vi "Process.vi"(8 "error in (no error)":errorcluster, 10 "Pound in":refnum<class "Pound.lvclass">, 11 "Qbus in":refnum<class "Qbus.lvclass">) -> (0 "error out":errorcluster)   [LabVIEW 2017, in "McsaFpgaAcquisition.lvlib"]
doc: "Acquires waveforms from channels on NI 9242 and NI 9239 C Series modules. This process transfers data from a device-specific FPGA bitfile that reads samples directly from the FPGA at the sampling rate configured for the device."
uses:
  <vilib>/addons/InsightCM/Devices/Shared/Mcsa/McsaFpgaAcquisition/McsaFpgaAcquisition.lvlib
  <vilib>/addons/Qbus/Qbus.lvclass
  <vilib>/NI/Software Watchdog/Pound/Pound.lvclass
  <vilib>/addons/InsightCM/Devices/Shared/Cms/CmsAcquisition/controls/State.ctl
  <vilib>/addons/InsightCM/Devices/Shared/Mcsa/McsaFpgaAcquisition/controls/Configuration.ctl
  <vilib>/addons/InsightCM/Devices/Shared/Cms/CmsAcquisition/controls/FixedSizeArrays.ctl
  <vilib>/LabVIEW Targets/FPGA/cRIO/shared/nicrio_ModuleControls/nicrio_cRIO-9232_ConfigModeRing.ctl
  <vilib>/addons/InsightCM/Devices/Shared/Cms/cRIOWfmAcq/subVIs/RIO Wfm Cust Ctrls/rwfm_SamplingInfo.ctl
  <vilib>/addons/InsightCM/Devices/Shared/Mcsa/McsaFpgaAcquisition/controls/Group.ctl
  <vilib>/addons/InsightCM/Devices/Shared/Mcsa/McsaFpgaAcquisition/controls/ChannelMcsa.ctl
  <vilib>/addons/InsightCM/Devices/Shared/Mcsa/McsaFpgaAcquisition/controls/RangeParams.ctl
  <vilib>/addons/InsightCM/Devices/Shared/Common/DataFlow/controls/Type.ctl
  <vilib>/addons/InsightCM/Devices/Shared/Cms/cRIOWfmAcq/cRIOWfmLib.lvlib
  <vilib>/NI/Software Watchdog/Watchdog/Watchdog.lvclass
  <vilib>/addons/InsightCM/Devices/Shared/Common/FpgaBitfileManager/FpgaBitfileManager.lvlib
  <vilib>/addons/InsightCM/Devices/Shared/Common/DataFlow/DataFlow.lvlib
  <vilib>/addons/InsightCM/Utilities/GlobalConfiguration/GlobalConfiguration.lvlib
  <vilib>/addons/InsightCM/Devices/Shared/Common/ServerComm/ServerComm.lvlib
  <vilib>/addons/InsightCM/Devices/Shared/Mcsa/cRIOWfmAcqMcsa/cRIOWfmLibMcsa.lvlib
  <vilib>/addons/InsightCM/Devices/Shared/Mcsa/McsaDataEventCreator/McsaDataEventCreator.lvlib
  <vilib>/addons/TraceLogger/TraceLogger.lvlib
  <vilib>/addons/InsightCM/Devices/Shared/Cms/CmsAcquisition/CmsAcquisition.lvlib
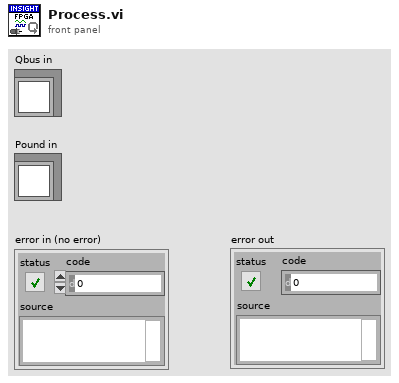
[diagram p1: front panel]
types:
  T1 = typedef "McsaFpgaAcquisition.lvlib/Configuration.ctl" = cluster{"NumberOfModules":i16, "Dynamic FPGA VI Ref":refnum<k20>, "FixedSizeX31":T2, "SamplingInfo":T4, "BlockSize (sec)":dbl, "Samples To Read (per chan)":i32, "RunningAcquisitionLength":dbl, "Settling Time":dbl, "Waveform Groups":T5[], "Acquisition Block Number":i32, "Device Name":string, "ValidConfig":bool, "delta connection?":bool}
  T2 = typedef "CmsAcquisition.lvlib/FixedSizeArrays.ctl" = cluster{"EnabledChannels":bool[], "Sensitivity":dbl[], "InputConfig":T3[]}
  T3 = typedef "nicrio_cRIO-9232_ConfigModeRing.ctl" = u8
  T4 = typedef "cRIOWfmLib.lvlib/rwfm_SamplingInfo.ctl" = cluster{"Number of Channels":i32, "Sampling Rate":dbl, "Channels":string[], "Units":string[], "Offsets":sgl[]}
  T5 = typedef "McsaFpgaAcquisition.lvlib/Group.ctl" = cluster{"Name":string, "Channels":T6[]}
  T6 = typedef "McsaFpgaAcquisition.lvlib/ChannelMcsa.ctl" = cluster{"Name":string, "Status Tag":string, "RangeCheck":T7}
  T7 = typedef "McsaFpgaAcquisition.lvlib/RangeParams.ctl" = cluster{"Enabled":bool, "Max":dbl, "Min":dbl}
  T8 = typedef "CmsAcquisition.lvlib/State.ctl" = enum16{"Unconfigured", "Configured", "Acquiring", "Stopped", "BurstMode"}
  T9 = typedef "DataFlow.lvlib/Type.ctl" = enum16{"High Rate", "Low Rate", "Burst Mode"}
  T10 = typedef "McsaDataEventCreator.lvlib/RegisterDataSets.ctl" = cluster{"DataGroup":string, "DataSets":T11[]}
  T11 = typedef "McsaDataEventCreator.lvlib/Registry_DataSet.ctl" = cluster{"ChannelName":string, "DataSetType":T12, "DoNotWriteToDB":bool, "ParentName":string}
  T12 = typedef "McsaDataEventCreator.lvlib/DataSetType.ctl" = enum16{"Waveform", "MCSAFFT", "TorqueWFM"}
  T13 = typedef "DataFlow.lvlib/Data.ctl" = cluster{"DataGroup":string, "Waveforms":T14, "Map":T15, "Type":T9}
  T14 = typedef "wfmSGL_DVR.ctl" = refnum<data-value>
  T15 = typedef "PointValueMap.lvlib/PointMap.ctl" = refnum<data-value>
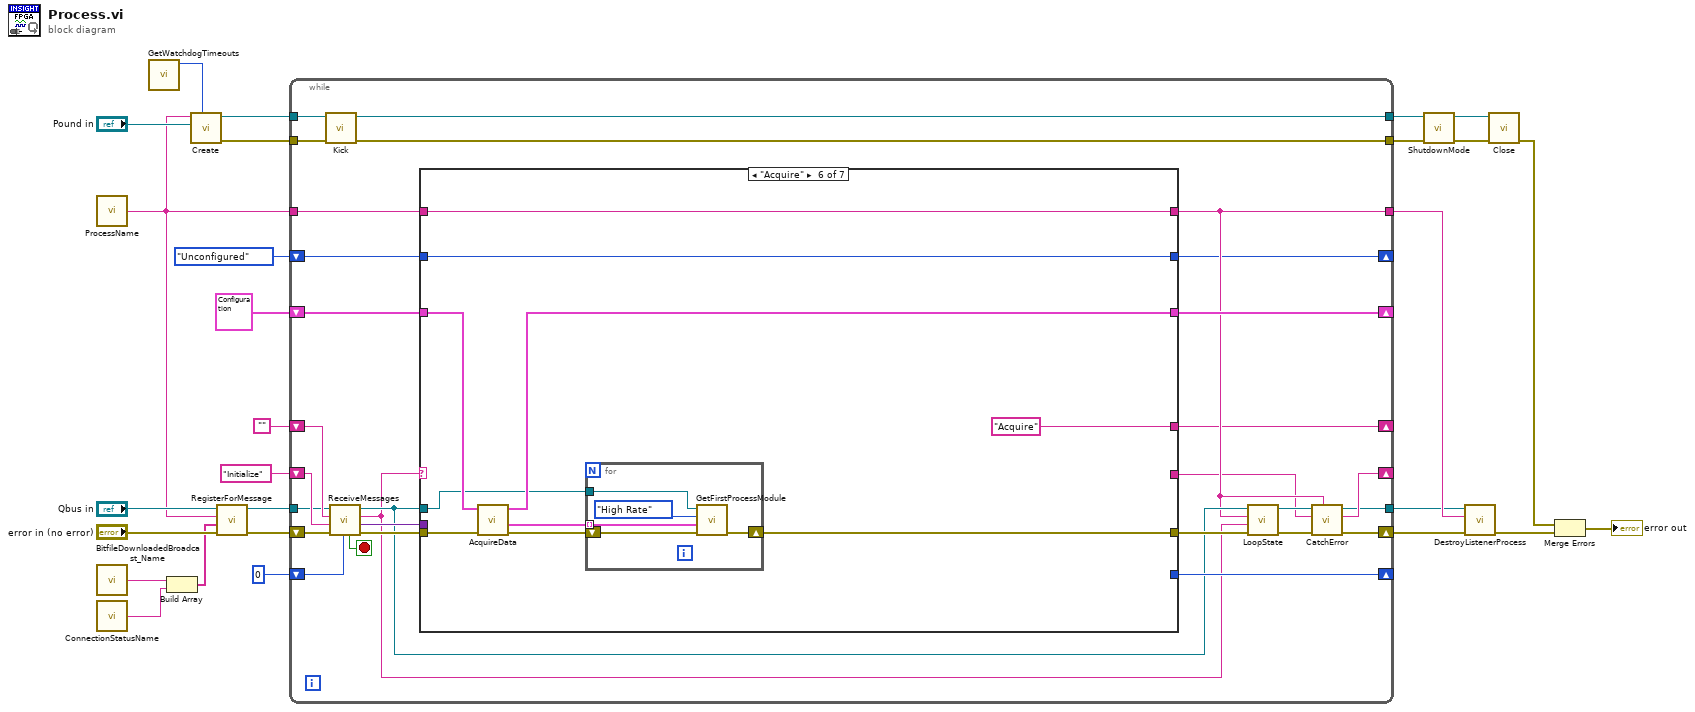
[diagram p0: block diagram]
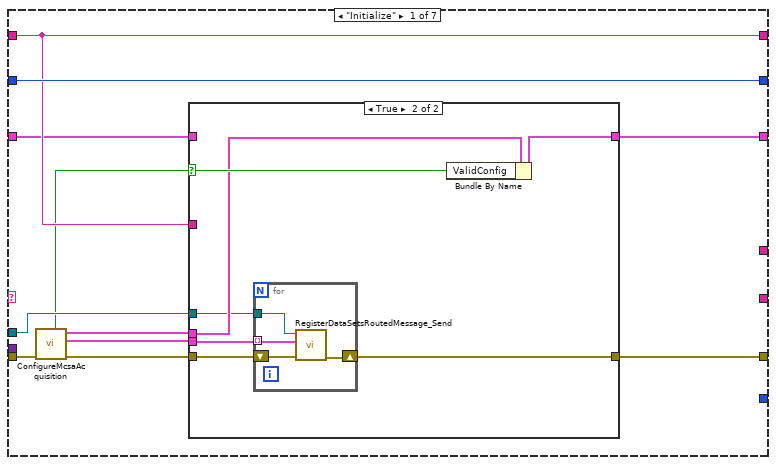
[diagram p2: hidden frame]
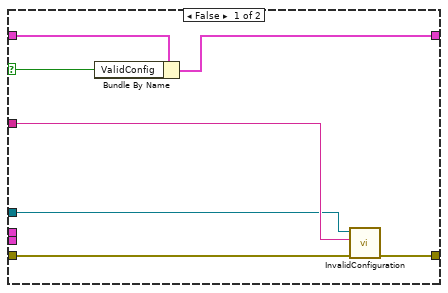
[diagram p3: hidden frame]
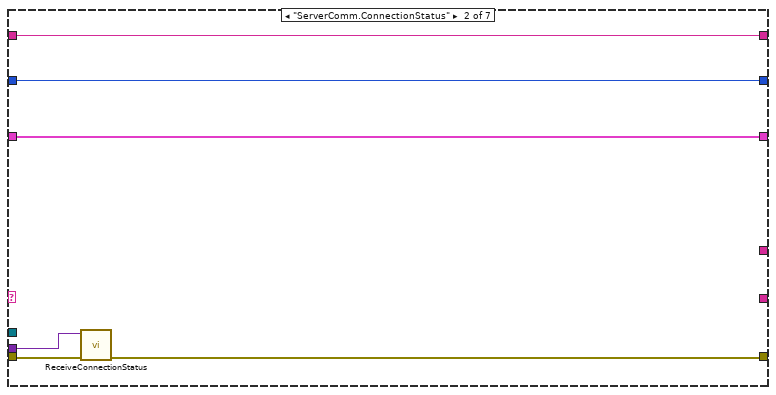
[diagram p4: hidden frame]
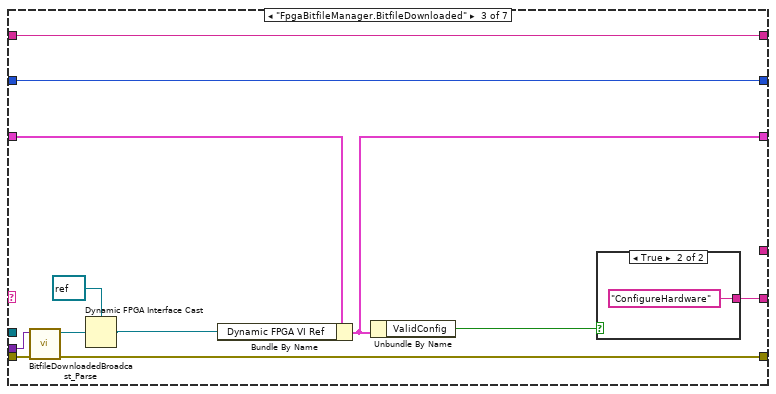
[diagram p5: hidden frame]
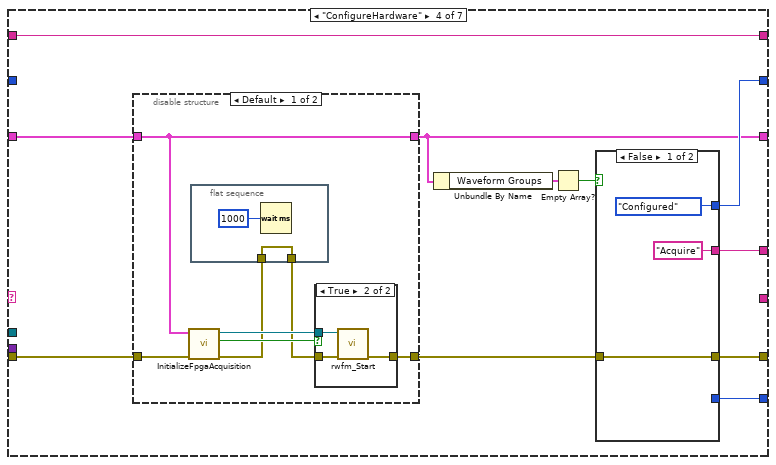
[diagram p7: hidden frame]
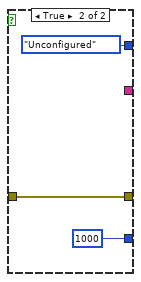
[diagram p8: hidden frame]
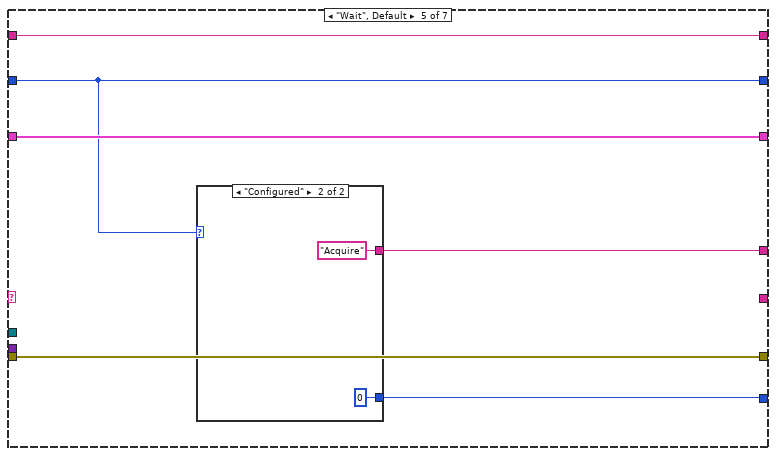
[diagram p11: hidden frame]
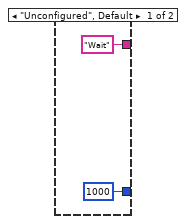
[diagram p12: hidden frame]
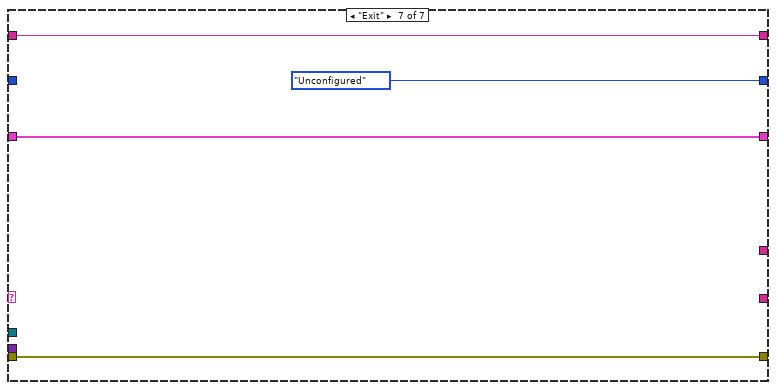
[diagram p13: hidden frame]
diagram:
  n1 = call <vilib>:"ProcessName.vi"() -> ("process name"=w4:string)  [unwired: 5 in]
  n2 = call <vilib>:"BitfileDownloadedBroadcast_Name.vi"() -> ("message name"=w9:string)  [unwired: 5 in]
  n3 = call <vilib>:"ConnectionStatusName.vi"() -> ("message name"=w1:string)  [unwired: 5 in]
  n4 = call <vilib>:"GetWatchdogTimeouts.vi"() -> ("software timeout"=w2:u32)  [unwired: 10 in, 1 out]
  n5 = Build Array(w9, w1) -> (w10:string[])
  n6 = call <vilib>:"Create.vi"("Execution Timeout (ms)"=w2, "Pound"="Pound in", "Name"=w4) -> ("error out"=w23:errorcluster, "Watchdog"=w24:refnum<data-value>)  [unwired: 7 in]
  n7 = call <vilib>:"RegisterForMessage.vi"("error in (no error)"="error in (no error)", "message names"=w10, "process name"=w4, "Qbus in"="Qbus in") -> ("error in (no error)"=w12:errorcluster, "Qbus out"=w13:refnum<class "Qbus.lvclass">)  [unwired: 6 in]
  n8 = while {
    shift-right: [w44] -> w5
    shift-left: w12 -> [w51]
    shift-right: [w34] -> _
    shift-left: "" -> [w53]
    shift-right: [w56] -> _
    shift-left: T1 {"NumberOfModules"=0, "Dynamic FPGA VI Ref"=refnum, "FixedSizeX31"={"EnabledChannels"=[], "Sensitivity"=[], "InputConfig"=[]}, "SamplingInfo"={"Number of Channels"=0, "Sampling Rate"=0.0, "Channels"=[], "Units"=[], "Offsets"=[]}, "BlockSize (sec)"=0.0, "Samples To Read (per chan)"=0, "RunningAcquisitionLength"=0.0, "Settling Time"=0.0, "Waveform Groups"=[], "Acquisition Block Number"=0, "Device Name"="", "ValidConfig"=FALSE, "delta connection?"=FALSE} ("MCSA Acquisition Configuration") -> [w28]
    shift-right: [w32] -> _
    shift-left: State."Unconfigured" ("loop state") -> [w55]
    shift-right: [w54] -> _
    shift-left: 0 ("milliseconds to wait") -> [w49]
    shift-right: [w42] -> _
    shift-left: "Initialize" -> [w52]
    tunnel: w13 -> [w50]
    tunnel: w4 -> [w29]
    tunnel: [w40] -> w6
    tunnel: [w35] -> w26
    tunnel: w24 -> [w39]
    tunnel: w23 -> [w38]
    tunnel: [w37] -> w20
    tunnel: [w36] -> w19
    stop <- w30 stop-if-true
    n9 = call <vilib>:"Kick.vi"("error in (no error)"=w38, "Watchdog"=w39) -> ("error out"=w36:errorcluster, "Watchdog"=w37:refnum<data-value>)  [unwired: 8 in]
    n10 = call <vilib>:"ReceiveMessages.vi"("timeout(100)"=w49, "error in (no error)"=w51, "priority action"=w52, "default action"=w53, "qbus in"=w50) -> ("error out"=w48:errorcluster, "msg value"=w47:variant, "action"=w31:string, "qbus out"=w43:refnum<class "Qbus.lvclass">, "exit"=w30:bool)  [unwired: 2 in]
    n11 = case shown="\"Acquire\"" w31 {
      tunnel: w48 -> [w65 w90 w95 w114 w142 w149 w162]
      tunnel: [w62 w89 w94 w111 w142 w148 w162] -> w45
      tunnel: [_ _ _ w110 w140 "Acquire" _] -> w34
      tunnel: [w57 w86 w93 w106 w141 w152 w165] -> w56
      tunnel: w28 -> [w58 w86 w102 w115 w141 w153 w165]
      tunnel: w55 -> [w63 w88 w98 _ w137 w151 _]
      tunnel: [_ _ _ w105 w138 _ _] -> w54
      tunnel: w29 -> [w60 w91 w103 w113 w139 w150 w163]
      tunnel: w47 -> [_ w87 w96 _ _ _ _]
      tunnel: w43 -> [w64 _ _ _ _ w147 _]
      tunnel: [w60 w91 w103 w113 w139 w150 w163] -> w35
      tunnel: [_ _ w99 _ _ _ _] -> w33
      tunnel: [w63 w88 w98 w109 w137 w151 State."Unconfigured" ("loop state")] -> w32
      frame "Initialize" {
        n12 = call <vilib>:"ConfigureMcsaAcquisition.vi"("error in (no error)"=w65) -> ("error out"=w67:errorcluster, "register data sets"=w66:T10[], "Mcsa Acquisition Config"=w61:T1, "valid"=w59:bool)  [unwired: 7 in]
        n13 = case shown="True" w59 {
          selector: w59 -> [w70 w77]
          tunnel: w67 -> [w68 w81]
          tunnel: w66 -> [_ w80]
          tunnel: w64 -> [w69 w75]
          tunnel: [w74 w79] -> w62
          tunnel: w61 -> [_ w76]
          tunnel: w60 -> [w73 _]
          tunnel: w58 -> [w72 _]
          tunnel: [w71 w78] -> w57
          frame False {
            n14 = Bundle By Name(cluster=w72, "ValidConfig"=w70) -> (w71:T1)
            n15 = call <vilib>:"InvalidConfiguration.vi"("error in (no error)"=w68, "description"=w73, "Qbus in"=w69) -> ("error out"=w74:errorcluster)  [unwired: 7 in, 1 out]
          }
          frame True {
            n16 = for {
              shift-right: [w84] -> w79
              shift-left: w81 -> [w85]
              tunnel: w80 -> [w82] mode=indexing
              tunnel: w75 -> [w83]
              n17 = call <vilib>:"RegisterDataSetsRoutedMessage_Send.vi"("error in (no error)"=w85, "RegisterDataSet"=w82, "Qbus in"=w83) -> ("error out"=w84:errorcluster)  [unwired: 7 in, 1 out]
            }
            n18 = Bundle By Name(cluster=w76, "ValidConfig"=w77) -> (w78:T1)
          }
        }
      }
      frame "ServerComm.ConnectionStatus" {
        n19 = call <vilib>:"ReceiveConnectionStatus.vi"("error in (no error)"=w90, "body"=w87) -> ("error out"=w89:errorcluster)  [unwired: 6 in, 3 out]
      }
      frame "FpgaBitfileManager.BitfileDownloaded" {
        n20 = call <vilib>:"BitfileDownloadedBroadcast_Parse.vi"("error in (no error)"=w95, "data"=w96) -> ("error out"=w94:errorcluster, "FPGA reference"=w97:refnum<k20>)  [unwired: 8 in]
        n21 = Dynamic FPGA Interface Cast(Session In=refnum<k20> refnum ("Dynamic FPGA VI Ref"), Type=w97) -> (Session Out=w101:refnum<k20>)
        n22 = Bundle By Name(cluster=w102, "Dynamic FPGA VI Ref"=w101) -> (w93:T1)
        n23 = Unbundle By Name(w93) -> ("ValidConfig"=w92:bool)
        n24 = case shown="True" w92 {
          tunnel: [_ "ConfigureHardware"] -> w99
          frame False {
          }
          frame True {
          }
        }
      }
      frame "ConfigureHardware" {
        n25 = disable-structure shown="Default" {
          disable-tunnel: w115 -> [w125 w135]
          disable-tunnel: w114 -> [w128 w136]
          disable-tunnel: [w127 w136] -> w112
          disable-tunnel: [w125 w135] -> w106
          frame condition #0 (active) {
            n26 = call <vilib>:"InitializeFpgaAcquisition.vi"("error in (no error)"=w128, "MCSA Acquisition Config"=w125) -> ("error out"=w123:errorcluster, "start acquisition?"=w124:bool, "dynamic FPGA VI reference"=w126:refnum<k20>)  [unwired: 7 in]
            n27 = flat-sequence {
              tunnel: [w129] -> w122
              tunnel: w123 -> [w129]
              frame #0 {
                n28 = Wait (ms)(milliseconds to wait=u32 1000) -> ()  [unwired: 1 out]
              }
            }
            n29 = case shown="True" w124 {
              tunnel: [w131 w134] -> w127
              tunnel: w122 -> [w131 w133]
              tunnel: w126 -> [_ w132]
              frame False {
              }
              frame True {
                n30 = call <vilib>:"rwfm_Start.vi"("error in"=w133, "Dynamic FPGA VI Reference"=w132) -> ("error out"=w134:errorcluster)  [unwired: 7 in, 2 out]
              }
            }
          }
          frame condition #1 {
            # "user could add simulated hardware here for MCSA device"
          }
        }
        n31 = Unbundle By Name(w106) -> ("Waveform Groups"=w108:T5[])
        n32 = Empty Array?(array=w108) -> (empty?=w107:bool)
        n33 = case shown="False" w107 {
          tunnel: ["Acquire" _] -> w110
          tunnel: [w117 w121] -> w111
          tunnel: w112 -> [w117 w121]
          tunnel: [_ 1000] -> w105
          tunnel: [State."Configured" ("loop state") State."Unconfigured" ("loop state")] -> w109
          frame False {
          }
          frame True {
          }
        }
      }
      frame "Wait", Default {
        n34 = case shown="\"Configured\"" w137 {
          tunnel: ["Wait" "Acquire"] -> w140
          tunnel: [1000 0] -> w138
          frame "Unconfigured", Default {
          }
          frame "Configured" {
          }
        }
      }
      frame "Acquire" {
        n35 = call <vilib>:"AcquireData.vi"("error in (no error)"=w149, "MCSA acquisition config"=w153) -> ("error out"=w155:errorcluster, "dataflow messages"=w154:T13[], "MCSA acquisition config out"=w152:T1)  [unwired: 7 in]
        n36 = for {
          tunnel: w154 -> [w158] mode=indexing
          tunnel: w147 -> [w159]
          shift-right: [w160] -> w148
          shift-left: w155 -> [w161]
          n37 = call <vilib>:"GetFirstProcessModule.vi"("error in (no error)"=w161, "data"=w158, "type"=Type."High Rate", "Qbus in"=w159) -> ("error out"=w160:errorcluster)  [unwired: 6 in, 1 out]
        }
      }
      frame "Exit" {
      }
    }
    n38 = call <vilib>:"LoopState.vi"("error in (no error)"=w45, "loop action"=w31, "process name"=w35, "Qbus in"=w43) -> ("error out"=w46:errorcluster, "Qbus out"=w41:refnum<class "Qbus.lvclass">)  [unwired: 6 in]
    n39 = call <vilib>:"CatchError.vi"("source"=w35, "error in (no error)"=w46, "next action in"=w33, "Qbus in"=w41) -> ("error out"=w44:errorcluster, "next action out"=w42:string, "Qbus out"=w40:refnum<class "Qbus.lvclass">)  [unwired: 5 in]
  }
  n40 = call <vilib>:"ShutdownMode.vi"("error in (no error)"=w19, "Watchdog"=w20) -> ("error out"=w21:errorcluster, "Watchdog"=w22:refnum<data-value>)  [unwired: 8 in]
  n41 = call <vilib>:"DestroyListenerProcess.vi"("error in (no error)"=w5, "process name"=w26, "Qbus in"=w6) -> ("error in (no error)"=w17:errorcluster)  [unwired: 7 in, 1 out]
  n42 = call <vilib>:"Close.vi"("error in (no error)"=w21, "Watchdog"=w22) -> ("error out"=w16:errorcluster)  [unwired: 9 in]
  n43 = Merge Errors(w16, w17) -> (→"error out":errorcluster)
